vi "roi profile by akram.vi"() -> ()   [LabVIEW 2011]
uses:
  <vilib>/vision/NI_Vision_Development_Module.lvlib
panel:
  out "error out":errorcluster
  out "ROI Pixel Statistics":T1 {"Min" format="%.2f"; "Std Dev" format="%.2f"; "Mean" format="%.2f"; "Max" format="%.2f"}
  out "Waveform Graph":sgl[](graph)
  out "Image":T2(plugin-control)
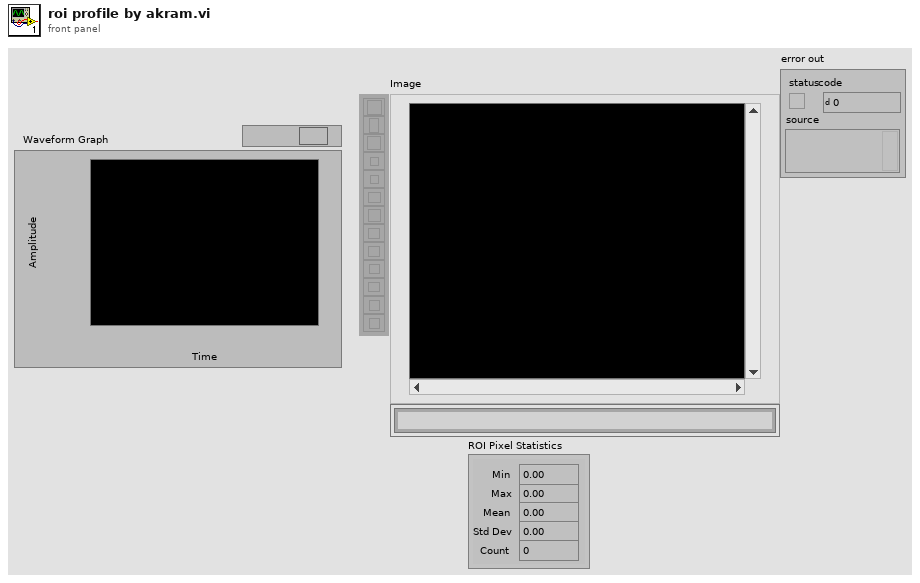
[diagram p1: front panel]
types:
  T1 = cluster{"Min":sgl, "Max":sgl, "Mean":sgl, "Std Dev":sgl, "Count":i32}
  T2 = typedef "IMAQ Image.ctl" = refnum<image>
  T3 = enum32{"AutoM", "Close", "Dilate", "Erode", "Gradient", "Gradient in", "Gradient out", "HitMiss", "Open", "PClose", "POpen", "Thick", "Thin"}
  T4 = typedef "ROI Descriptor" = cluster{"Global Rectangle":i32[], "Contours":cluster{"ID":enum32{"External", "Internal"}, "Type":u32, "Coordinates":i32[]}[]}
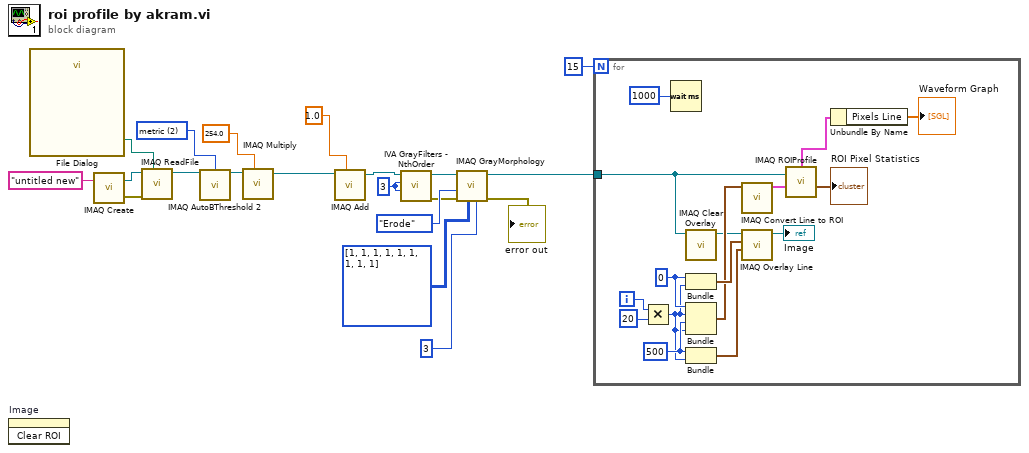
[diagram p0: block diagram]
diagram:
  w9 = 3 ("Filter size X")
  w14 = 2 items=["clustering", "entropy", "metric", "moments", "inter-class variance"] ("Method (clustering)")
  n1 = invoke on="Image" class="ImageControl" method="Clear ROI"() -> ()  [unwired: 3 in, 3 out]
  n2 = call "File Dialog"() -> ("selected path"=w17:path)  [unwired: 12 in, 3 out]
  n3 = call "IMAQ Create"("Image Name"="untitled new") -> ("New Image"=w18:T2, "error out"=w19:errorcluster)  [unwired: 4 in]
  n4 = call "IMAQ ReadFile"("File Path"=w17, "error in (no error)"=w19, "Image"=w18) -> ("Image Out"=w15:T2)  [unwired: 4 in, 4 out]
  n5 = call "IMAQ AutoBThreshold 2"("Image Src"=w15, "Method (clustering)"=w14) -> ("Image Dst Out"=w13:T2)  [unwired: 6 in, 7 out]
  n6 = call "IMAQ Multiply"("Image Src A"=w13, "Constant"=sgl 254.0) -> ("Image Dst Out"=w10:T2)  [unwired: 5 in, 1 out]
  n7 = call "IMAQ Add"("Image Src A"=w10, "Constant"=sgl 1.0) -> ("Image Dst Out"=w2:T2)  [unwired: 5 in, 1 out]
  n8 = call <vilib>:"IVA GrayFilters - NthOrder.vi"("Filter size Y"=w9, "Filter size X"=w9, "Image In"=w2) -> ("error out"=w4:errorcluster, "Image Out"=w6:T2)  [unwired: 1 in, 6 out]
  n9 = call "IMAQ GrayMorphology"("Number of iterations (1)"=3, "Structuring Element"=i32[][] [[1, 1, 1], [1, 1, 1], [1, 1, 1]] ("Structuring Element (Gray Morphology 1)"), "error in (no error)"=w4, "Operation"=T3."Erode" ("Operation (Gray Morphology 1)"), "Image Src"=w6) -> ("error out"=→"error out":errorcluster, "Image Dst Out"=w1:T2)  [unwired: 2 in, 3 out]
  n10 = for {
    N: 15 -> [_]
    tunnel: w1 -> [w24]
    i -> [w30]
    w31 = 500 ("End Y")
    w32 = 0 ("End Y")
    n11 = Multiply(x=w30, y=20) -> (x*y=w27:i32)
    n12 = Wait (ms)(milliseconds to wait=u32 1000) -> ()  [unwired: 1 out]
    n13 = call "IMAQ Clear Overlay"("Image"=w24) -> ("Image Out"=w22:T2)  [unwired: 9 in, 1 out]
    n14 = Bundle("End Y"=w32, w27) -> (w36:cluster{"End Y":i32, i32})  [unwired: 1 in]
    n15 = Bundle("End Y"=w32, w27, "End Y"=w31, w27) -> (w29:cluster{"End Y":i32, i32, "End Y":i32, i32})  [unwired: 1 in]
    n16 = Bundle("End Y"=w31, w27) -> (w35:cluster{"End Y":i32, i32})  [unwired: 1 in]
    n17 = call "IMAQ Convert Line to ROI"("Line"=w29) -> ("ROI Descriptor"=w28:T4)  [unwired: 8 in, 1 out]
    n18 = call "IMAQ Overlay Line"("End Point"=w35, "Start Point"=w36, "Image"=w22) -> ("Image Out"=→"Image":T2)  [unwired: 7 in, 1 out]
    n19 = call "IMAQ ROIProfile"("ROI Descriptor"=w28, "Image"=w24) -> ("ROI Pixel Statistics"=→"ROI Pixel Statistics":T1, "ROI Graph"=w33:cluster{"x0":sgl, "dx":sgl, "Pixels Line":sgl[]})  [unwired: 2 in, 3 out]
    n20 = Unbundle By Name(w33) -> ("Pixels Line"=→"Waveform Graph":sgl[])
  }
